vi "New Folder.vi"(8 "error in (no error)":errorcluster, 10 "Folder (\"INT:\\new\")":string="INT:\\new", 11 "VISA resource name":refnum<visa-resource-name>) -> (0 "error out":errorcluster, 3 "VISA resource name out":refnum<visa-resource-name>)   [LabVIEW 2020, in "AWG.lvlib" / "Agilent 3352X Series.lvlib"]
doc: "Makes a new directory (folder) at the specified location of the file path on the mass storage ( the instrument memory or an external USB memory)"
uses:
  Agilent 3352X Series.lvlib
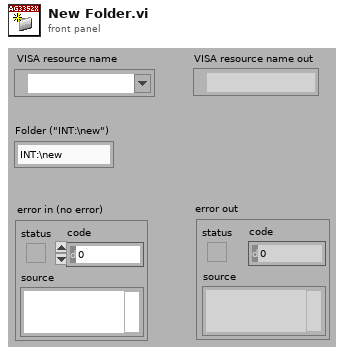
[diagram p1: front panel]
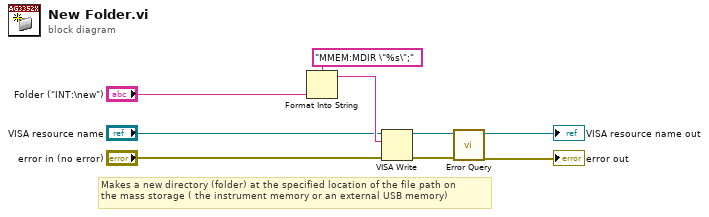
[diagram p0: block diagram]
diagram:
  # "Makes a new directory (folder) at the specified location of the file path on \nthe mass storage ( the instrument memory or an external USB memory)"
  n1 = Format Into String(format string="MMEM:MDIR \"%s\";", "Folder (\"INT:\\new\")") -> (resulting string=w8:string)  [unwired: 2 in, 1 out]
  n2 = VISA Write(VISA resource name="VISA resource name", write buffer=w8, error in (no error)="error in (no error)") -> (VISA resource name out=w5:refnum<visa-resource-name>, error out=w4:errorcluster)  [unwired: 1 out]
  n3 = call "Error Query.vi"("error in (no error)"=w4, "VISA resource name"=w5) -> ("error out"=→"error out":errorcluster, "VISA resource name out"=→"VISA resource name out":refnum<visa-resource-name>)  [unwired: 8 out]
